vi "Read Passed count.vi"(11 "Test Suite Result In":refnum<class "Test Suite Result.lvclass">) -> (2 "Pass count":i32, 3 "Test Suite Result Out":refnum<class "Test Suite Result.lvclass">)   [LabVIEW 2020, in "Test Suite Result.lvclass"]
uses:
  Test Suite Result.lvclass
  Assertion Result/Public/TypeDefs/Status.ctl
  Test Suite Result.lvclass/Test Suite Result.ctl
  Test Case Result/Test Case Result.lvclass/Test Case Result.ctl
  Method Result/Method Result.lvclass/Method Result.ctl
  Test Case Result/Public/Accessors/Read Status.vi
  Test Case Result/Private/SubVIs/Merge Status.vi
  Method Result/Public/Read Status.vi
  Assertion Result/Assertion Result.lvclass
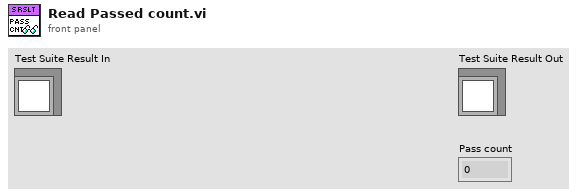
[diagram p1: front panel]
types:
  T1 = typedef "Assertion Result.lvclass/Status.ctl" = enum16{"Pass", "Fail", "Error", "Skipped", "Setup Error", "Broken", "Teardown Error"}
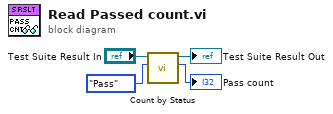
[diagram p0: block diagram]
diagram:
  n1 = call "Count by Status.vi"("Status"=Status."Pass", "Test Suite Result in"="Test Suite Result In") -> ("Count"=→"Pass count":i32, "Test Suite Result out"=→"Test Suite Result Out":refnum<class "Test Suite Result.lvclass">)  [unwired: 8 in]
